vi "Compile - Tx Packet Information.vi"(8 "error in (no error)":errorcluster, 11 "Custom Device Ref in":T1 format="%.0x") -> (0 "error out":errorcluster, 1 "Tx Ref Array":T2(array[cluster]) {"VS Refs" format="%.0x"}, 2 "Tx Packet Info Array":T3[](array[typedef]) {"Endianness" items=["big-endian"=0, "little-indian"=2]}, 3 "Custom Device Ref out":T1 format="%.0x")   [LabVIEW 2016, in "UDP-Custom-Device System Explorer.lvlib"]
uses:
  UDP-Custom-Device System Explorer.lvlib
  Shared/Types/Shared - Tx.PacketInfo.ctl
  Shared/Types/Shared - Channel Data Type.ctl
  Shared/Types/Shared - Header Details.ctl
  Shared/Types/Shared - Buffered.PacketInfo.ctl
  <vilib>/NI Veristand/Custom Device API/Custom Device Item Ref.ctl
  Shared/UDP-Custom-Device Shared.lvlib
  <vilib>/NI VeriStand/Custom Device API/Custom Device API.lvlib
  Property Accessors/Tx Packet Accessors.lvlib
  Property Accessors/Shared Packet Accessors.lvlib
  Property Accessors/Buffered Data Packet.lvlib
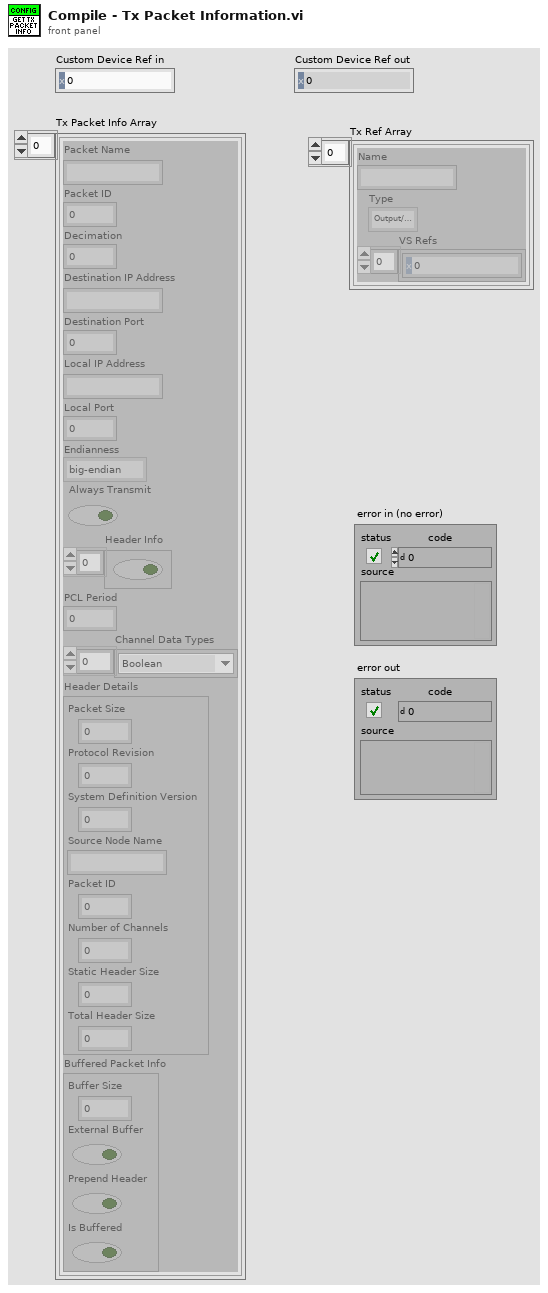
[diagram p1: front panel]
types:
  T1 = typedef "Custom Device API.lvlib/Custom Device Item Ref.ctl" = u64
  T2 = cluster{"Name":string, "Type":enum16{"Output/Write", "Input/Read", "Input/ReadWrite"}, "VS Refs":T1[]}[]
  T3 = typedef "UDP-Custom-Device Shared.lvlib/Shared - Tx.PacketInfo.ctl" = cluster{"Packet Name":string, "Packet ID":i32, "Decimation":u16, "Destination IP Address":string, "Destination Port":u16, "Local IP Address":string, "Local Port":u16, "Endianness":u16, "Always Transmit":bool, "Header Info":bool[], "PCL Period":u32, "Channel Data Types":T4[], "Header Details":T5, "Buffered Packet Info":T6}
  T4 = typedef "UDP-Custom-Device Shared.lvlib/Shared - Channel Data Type.ctl" = enum16{"Boolean", "Single", "Double", "I8", "I16", "I32", "I64", "U8", "U16", "U32", "U64"}
  T5 = typedef "UDP-Custom-Device Shared.lvlib/Shared - Header Details.ctl" = cluster{"Packet Size":u16, "Protocol Revision":u8, "System Definition Version":u64, "Source Node Name":string, "Packet ID":u32, "Number of Channels":u32, "Static Header Size":u16, "Total Header Size":u16}
  T6 = typedef "UDP-Custom-Device Shared.lvlib/Shared - Buffered.PacketInfo.ctl" = cluster{"Buffer Size":i32, "External Buffer":bool, "Prepend Header":bool, "Is Buffered":bool}
  T7 = typedef "UDP-Custom-Device System Explorer.lvlib/Packet Type.ctl" = enum16{"Transmit", "Receive", "Buffered Transmit", "Buffered Receive"}
  T8 = typedef "Custom Device API.lvlib/Custom Device Item Info.ctl" = cluster{"Name":string, "Is Channel":bool, "GUID":string, "Is Waveform":bool}
  T9 = cluster{"Name":string, "Type":enum16{"Output/Write", "Input/Read", "Input/ReadWrite"}, "VS Refs":T1[]}
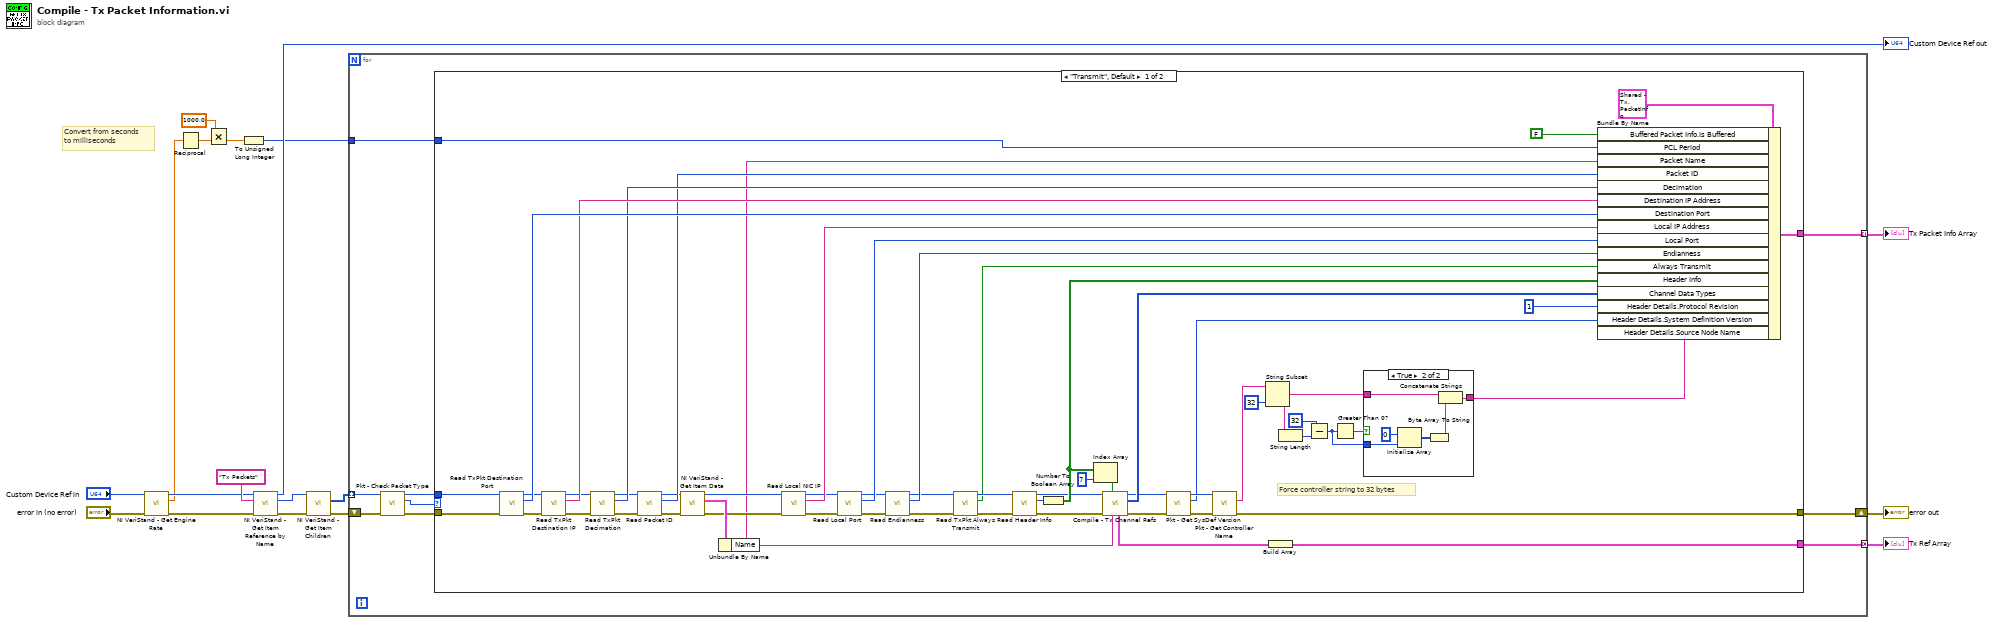
[diagram p0: block diagram]
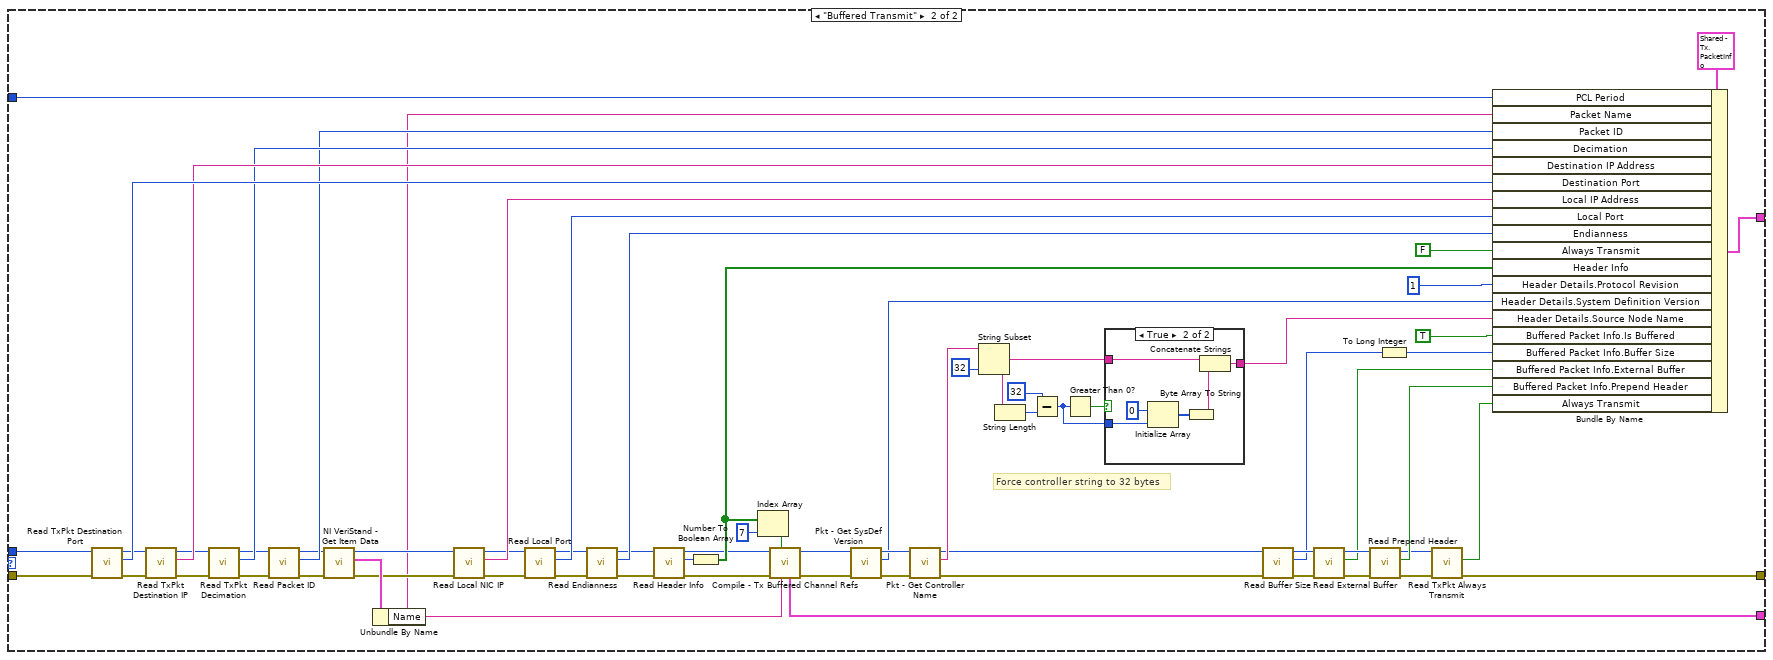
[diagram p3: hidden frame]
diagram:
  # "Convert from seconds\nto milliseconds"
  n1 = call <vilib>:"NI VeriStand - Get Engine Rate.vi"("error in (no error)"="error in (no error)", "Item Ref in"="Custom Device Ref in") -> ("error out"=w7:errorcluster, "Rate (Hz)"=w5:dbl, "Item Ref out"=w6:T1)  [unwired: 7 in]
  n2 = Reciprocal(x=w5) -> (1/x=w1:dbl)
  n3 = Multiply(x=1000.0, y=w1) -> (x*y=w3:dbl)
  n4 = To Unsigned Long Integer(number=w3) -> (unsigned 32bit integer=w4:u32)
  n5 = call <vilib>:"NI VeriStand - Get Item Reference by Name.vi"("error in (no error)"=w7, "Item Name"="Tx Packets", "Parent Ref in"=w6) -> ("error out"=w13:errorcluster, "Item Ref"=w11:T1, "Parent Ref out"=→"Custom Device Ref out":T1)  [unwired: 5 in, 1 out]
  n6 = call <vilib>:"NI VeriStand - Get Item Children.vi"("error in (no error)"=w13, "Item Ref in"=w11) -> ("error out"=w16:errorcluster, "Child Refs"=w15:T1[])  [unwired: 6 in, 2 out]
  n7 = for {
    shift-right: [w24] -> w18
    shift-left: w16 -> [w23]
    tunnel: [w27] -> w17 mode=indexing
    tunnel: w15 -> [w21] mode=indexing
    tunnel: [w25] -> w14 mode=concatenating
    tunnel: w4 -> [w26]
    n8 = call "Pkt - Check Packet Type.vi"("error in (no error)"=w23, "Node Ptr In"=w21) -> ("error out"=w22:errorcluster, "Packet Type"=w19:T7, "Node Ptr Out"=w20:T1)  [unwired: 7 in]
    n9 = case shown="\"Transmit\", Default" w19 {
      tunnel: [w84 w158] -> w27
      tunnel: w26 -> [w83 w157]
      tunnel: [w33 w98] -> w25
      tunnel: [w77 w93] -> w24
      tunnel: w20 -> [w63 w142]
      tunnel: w22 -> [w62 w141]
      frame "Transmit", Default {
        # "Force controller string to 32 bytes"
        n10 = call "Read TxPkt Destination Port.vi"("error in (no error)"=w62, "Node Ptr"=w63) -> ("error out"=w59:errorcluster, "Destination Port"=w61:u16, "Node Ptr out"=w60:T1)  [unwired: 7 in]
        n11 = call "Read TxPkt Destination IP.vi"("error in (no error)"=w59, "Node Ptr"=w60) -> ("error out"=w56:errorcluster, "Destination IP"=w58:string, "Node Ptr out"=w57:T1)  [unwired: 7 in]
        n12 = call "Read TxPkt Decimation.vi"("error in (no error)"=w56, "Node Ptr"=w57) -> ("error out"=w53:errorcluster, "Decimation"=w55:u16, "Node Ptr out"=w54:T1)  [unwired: 7 in]
        n13 = call "Read Packet ID.vi"("error in (no error)"=w53, "Node Ptr"=w54) -> ("error out"=w40:errorcluster, "Packet ID"=w52:i32, "Node Ptr out"=w41:T1)  [unwired: 7 in]
        n14 = call <vilib>:"NI VeriStand - Get Item Data.vi"("error in (no error)"=w40, "Item Ref in"=w41) -> ("error out"=w37:errorcluster, "Item Info"=w39:T8, "Item Ref out"=w38:T1)  [unwired: 6 in, 1 out]
        n15 = Unbundle By Name(w39) -> ("Name"=w36:string)
        n16 = call "Read Local NIC IP.vi"("error in (no error)"=w37, "Node Ptr"=w38) -> ("error out"=w49:errorcluster, "IP Address of Local NIC"=w51:string, "Node Ptr out"=w50:T1)  [unwired: 7 in]
        n17 = call "Read Local Port.vi"("error in (no error)"=w49, "Node Ptr"=w50) -> ("error out"=w46:errorcluster, "Port"=w48:u16, "Node Ptr out"=w47:T1)  [unwired: 7 in]
        n18 = call "Read Endianness.vi"("error in (no error)"=w46, "Node Ptr"=w47) -> ("error out"=w32:errorcluster, "Endianness"=w45:u16, "Node Ptr out"=w30:T1)  [unwired: 7 in]
        n19 = call "Read TxPkt Always Transmit.vi"("error in (no error)"=w32, "Node Ptr"=w30) -> ("error out"=w31:errorcluster, "Always Transmit?"=w28:bool, "Node Ptr out"=w29:T1)  [unwired: 7 in]
        n20 = call "Read Header Info.vi"("error in (no error)"=w31, "Node Ptr"=w29) -> ("error out"=w42:errorcluster, "Header Info"=w43:u32, "Node Ptr out"=w44:T1)  [unwired: 7 in]
        n21 = Number To Boolean Array(number=w43) -> (Boolean array=w81:bool[])
        n22 = Index Array(array=w81, index=7) -> (element=w79:bool)
        n23 = call "Compile - Tx Channel Refs.vi"("Packet Name"=w36, "Timestamp Present?"=w79, "error in (no error)"=w42, "Item Ref in"=w44) -> ("error out"=w66:errorcluster, "Data types"=w78:T4[], "Item Ref out"=w68:T1, "Tx Ref Array"=w34:T9)  [unwired: 4 in]
        n24 = call "Pkt - Get SysDef Version.vi"("error in (no error)"=w66, "Packet Ref In"=w68) -> ("error out"=w65:errorcluster, "Encoded Version"=w64:u64, "Packet Ref out"=w67:T1)  [unwired: 6 in, 1 out]
        n25 = call "Pkt - Get Controller Name.vi"("error in (no error)"=w65, "Packet Ref In"=w67) -> ("error out"=w77:errorcluster, "Name"=w76:string)  [unwired: 7 in, 1 out]
        n26 = String Subset(string=w76, length (rest)=32 ("length (rest)")) -> (substring=w70:string)  [unwired: 1 in]
        n27 = Build Array(w34) -> (w33:T2)
        n28 = String Length(string=w70) -> (length=w73:i32)
        n29 = Subtract(x=32 ("length (rest)"), y=w73) -> (x-y=w71:i32)
        n30 = Greater Than 0?(x=w71) -> (x > 0?=w72:bool)
        n31 = case shown="True" w72 {
          tunnel: w71 -> [_ w92]
          tunnel: w70 -> [w86 w89]
          tunnel: [w86 w87] -> w69
          frame False {
          }
          frame True {
            n32 = Initialize Array(u8 0, w92) -> (w90:u8[])
            n33 = Byte Array To String(unsigned byte array=w90) -> (string=w88:string)
            n34 = Concatenate Strings(w89, w88) -> (w87:string)
          }
        }
        n35 = Bundle By Name(cluster=T3 {"Packet Name"="", "Packet ID"=0, "Decimation"=0, "Destination IP Address"="", "Destination Port"=0, "Local IP Address"="", "Local Port"=0, "Endianness"=0, "Always Transmit"=FALSE, "Header Info"=[], "PCL Period"=0, "Channel Data Types"=[], "Header Details"={"Packet Size"=0, "Protocol Revision"=0, "System Definition Version"=0, "Source Node Name"="", "Packet ID"=0, "Number of Channels"=0, "Static Header Size"=0, "Total Header Size"=0}, "Buffered Packet Info"={"Buffer Size"=0, "External Buffer"=FALSE, "Prepend Header"=FALSE, "Is Buffered"=FALSE}} ("Packet Info"), "Buffered Packet Info.Is Buffered"=FALSE, "PCL Period"=w83, "Packet Name"=w36, "Packet ID"=w52, "Decimation"=w55, "Destination IP Address"=w58, "Destination Port"=w61, "Local IP Address"=w51, "Local Port"=w48, "Endianness"=w45, "Always Transmit"=w28, "Header Info"=w81, "Channel Data Types"=w78, "Header Details.Protocol Revision"=u8 1, "Header Details.System Definition Version"=w64, "Header Details.Source Node Name"=w69) -> (w84:T3)
      }
      frame "Buffered Transmit" {
        # "Force controller string to 32 bytes"
        n36 = call "Read TxPkt Destination Port.vi"("error in (no error)"=w141, "Node Ptr"=w142) -> ("error out"=w138:errorcluster, "Destination Port"=w140:u16, "Node Ptr out"=w139:T1)  [unwired: 7 in]
        n37 = call "Read TxPkt Destination IP.vi"("error in (no error)"=w138, "Node Ptr"=w139) -> ("error out"=w135:errorcluster, "Destination IP"=w137:string, "Node Ptr out"=w136:T1)  [unwired: 7 in]
        n38 = call "Read TxPkt Decimation.vi"("error in (no error)"=w135, "Node Ptr"=w136) -> ("error out"=w132:errorcluster, "Decimation"=w134:u16, "Node Ptr out"=w133:T1)  [unwired: 7 in]
        n39 = call "Read Packet ID.vi"("error in (no error)"=w132, "Node Ptr"=w133) -> ("error out"=w121:errorcluster, "Packet ID"=w131:i32, "Node Ptr out"=w122:T1)  [unwired: 7 in]
        n40 = call <vilib>:"NI VeriStand - Get Item Data.vi"("error in (no error)"=w121, "Item Ref in"=w122) -> ("error out"=w118:errorcluster, "Item Info"=w120:T8, "Item Ref out"=w119:T1)  [unwired: 6 in, 1 out]
        n41 = Unbundle By Name(w120) -> ("Name"=w99:string)
        n42 = call "Read Local NIC IP.vi"("error in (no error)"=w118, "Node Ptr"=w119) -> ("error out"=w128:errorcluster, "IP Address of Local NIC"=w130:string, "Node Ptr out"=w129:T1)  [unwired: 7 in]
        n43 = call "Read Local Port.vi"("error in (no error)"=w128, "Node Ptr"=w129) -> ("error out"=w125:errorcluster, "Port"=w127:u16, "Node Ptr out"=w126:T1)  [unwired: 7 in]
        n44 = call "Read Endianness.vi"("error in (no error)"=w125, "Node Ptr"=w126) -> ("error out"=w115:errorcluster, "Endianness"=w124:u16, "Node Ptr out"=w116:T1)  [unwired: 7 in]
        n45 = call "Read Header Info.vi"("error in (no error)"=w115, "Node Ptr"=w116) -> ("error out"=w102:errorcluster, "Header Info"=w123:u32, "Node Ptr out"=w103:T1)  [unwired: 7 in]
        n46 = Number To Boolean Array(number=w123) -> (Boolean array=w155:bool[])
        n47 = Index Array(array=w155, index=7) -> (element=w104:bool)
        n48 = call "Compile - Tx Buffered Channel Refs.vi"("Packet Name"=w99, "Timestamp Present?"=w104, "error in (no error)"=w102, "Item Ref in"=w103) -> ("error out"=w100:errorcluster, "Item Ref out"=w101:T1, "Tx Ref Array"=w98:T2)  [unwired: 5 in]
        n49 = call "Pkt - Get SysDef Version.vi"("error in (no error)"=w100, "Packet Ref In"=w101) -> ("error out"=w144:errorcluster, "Encoded Version"=w143:u64, "Packet Ref out"=w145:T1)  [unwired: 6 in, 1 out]
        n50 = call "Pkt - Get Controller Name.vi"("error in (no error)"=w144, "Packet Ref In"=w145) -> ("error out"=w108:errorcluster, "Name"=w153:string, "Packet Ref out"=w113:T1)  [unwired: 7 in]
        n51 = String Subset(string=w153, length (rest)=32 ("length (rest)")) -> (substring=w147:string)  [unwired: 1 in]
        n52 = String Length(string=w147) -> (length=w150:i32)
        n53 = Subtract(x=32 ("length (rest)"), y=w150) -> (x-y=w148:i32)
        n54 = Greater Than 0?(x=w148) -> (x > 0?=w149:bool)
        n55 = case shown="True" w149 {
          tunnel: w148 -> [_ w166]
          tunnel: w147 -> [w160 w163]
          tunnel: [w160 w161] -> w146
          frame False {
          }
          frame True {
            n56 = Initialize Array(u8 0, w166) -> (w164:u8[])
            n57 = Byte Array To String(unsigned byte array=w164) -> (string=w162:string)
            n58 = Concatenate Strings(w163, w162) -> (w161:string)
          }
        }
        n59 = call "Read Buffer Size.vi"("error in (no error)"=w108, "Node Ptr"=w113) -> ("error out"=w110:errorcluster, "Buffer Size"=w107:u32, "Node Ptr out"=w112:T1)  [unwired: 7 in]
        n60 = call "Read External Buffer.vi"("error in (no error)"=w110, "Node Ptr"=w112) -> ("error out"=w109:errorcluster, "External Buffer"=w106:bool, "Node Ptr out"=w111:T1)  [unwired: 7 in]
        n61 = call "Read Prepend Header.vi"("error in (no error)"=w109, "Node Ptr"=w111) -> ("error out"=w94:errorcluster, "Prepend Header"=w105:bool, "Node Ptr out"=w96:T1)  [unwired: 7 in]
        n62 = To Long Integer(number=w107) -> (32bit integer=w97:i32)
        n63 = call "Read TxPkt Always Transmit.vi"("error in (no error)"=w94, "Node Ptr"=w96) -> ("error out"=w93:errorcluster, "Always Transmit?"=w95:bool)  [unwired: 7 in, 1 out]
        n64 = Bundle By Name(cluster=T3 {"Packet Name"="", "Packet ID"=0, "Decimation"=0, "Destination IP Address"="", "Destination Port"=0, "Local IP Address"="", "Local Port"=0, "Endianness"=0, "Always Transmit"=FALSE, "Header Info"=[], "PCL Period"=0, "Channel Data Types"=[], "Header Details"={"Packet Size"=0, "Protocol Revision"=0, "System Definition Version"=0, "Source Node Name"="", "Packet ID"=0, "Number of Channels"=0, "Static Header Size"=0, "Total Header Size"=0}, "Buffered Packet Info"={"Buffer Size"=0, "External Buffer"=FALSE, "Prepend Header"=FALSE, "Is Buffered"=FALSE}} ("Packet Info"), "PCL Period"=w157, "Packet Name"=w99, "Packet ID"=w131, "Decimation"=w134, "Destination IP Address"=w137, "Destination Port"=w140, "Local IP Address"=w130, "Local Port"=w127, "Endianness"=w124, "Always Transmit"=FALSE ("Diagnostics En?"), "Header Info"=w155, "Header Details.Protocol Revision"=u8 1, "Header Details.System Definition Version"=w143, "Header Details.Source Node Name"=w146, "Buffered Packet Info.Is Buffered"=TRUE, "Buffered Packet Info.Buffer Size"=w97, "Buffered Packet Info.External Buffer"=w106, "Buffered Packet Info.Prepend Header"=w105, "Always Transmit"=w95) -> (w158:T3)
      }
    }
  }
  "Tx Packet Info Array" <- w17
  "error out" <- w18
  "Tx Ref Array" <- w14
